vi "Zad2.vi"() -> ()   [LabVIEW 2017]
uses:
  <vilib>/sound2/lvsound2.llb/Sound Data Format.ctl
  Lab 6 - 9.04.2018/mainVIs/States.ctl
  <vilib>/sound2/lvsound2.llb/Sound Input Task ID.ctl
  main VIs/UIData.ctl
  <vilib>/sound2/lvsound2.llb/Sampling Mode.ctl
  <vilib>/measure/maspectr.llb/FFT Power Spectrum and PSD for N Chan.vi
  <vilib>/sound2/lvsound2.llb/Sound Input Read (DBL).vi
  <vilib>/measure/NI_MAPro.lvlib
panel:
  out "Waveform Graph":cluster{"f0":dbl, "df":dbl, "magnitude":dbl[]}[](graph)
  in  "Stop":bool
  in  "Play":bool
  in  "sound format":T1={"sample rate (S/s)"=22050.0, "number of channels"=2, "bits per sample"=16}
  in  "number of samples/ch":i32=100000
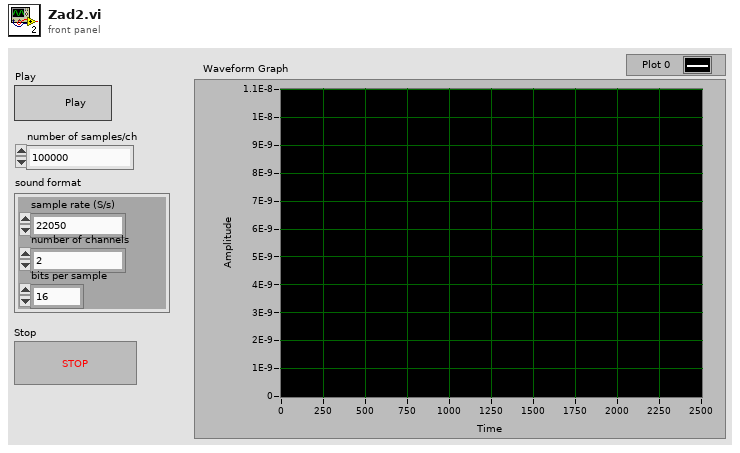
[diagram p1: front panel]
types:
  T1 = typedef "Sound Data Format.ctl" = cluster{"sample rate (S/s)":dbl, "number of channels":i32, "bits per sample":i32}
  T2 = typedef "Sound Input Task ID.ctl" = u32
  T3 = typedef "States.ctl" = enum16{"Idle", "Initialization", "Acquisition", "Finish"}
  T4 = typedef "UIData.ctl" = cluster{"Play":bool, "number of samples/ch":i32, "sound format":T1}
  T5 = typedef "Sampling Mode.ctl" = i32
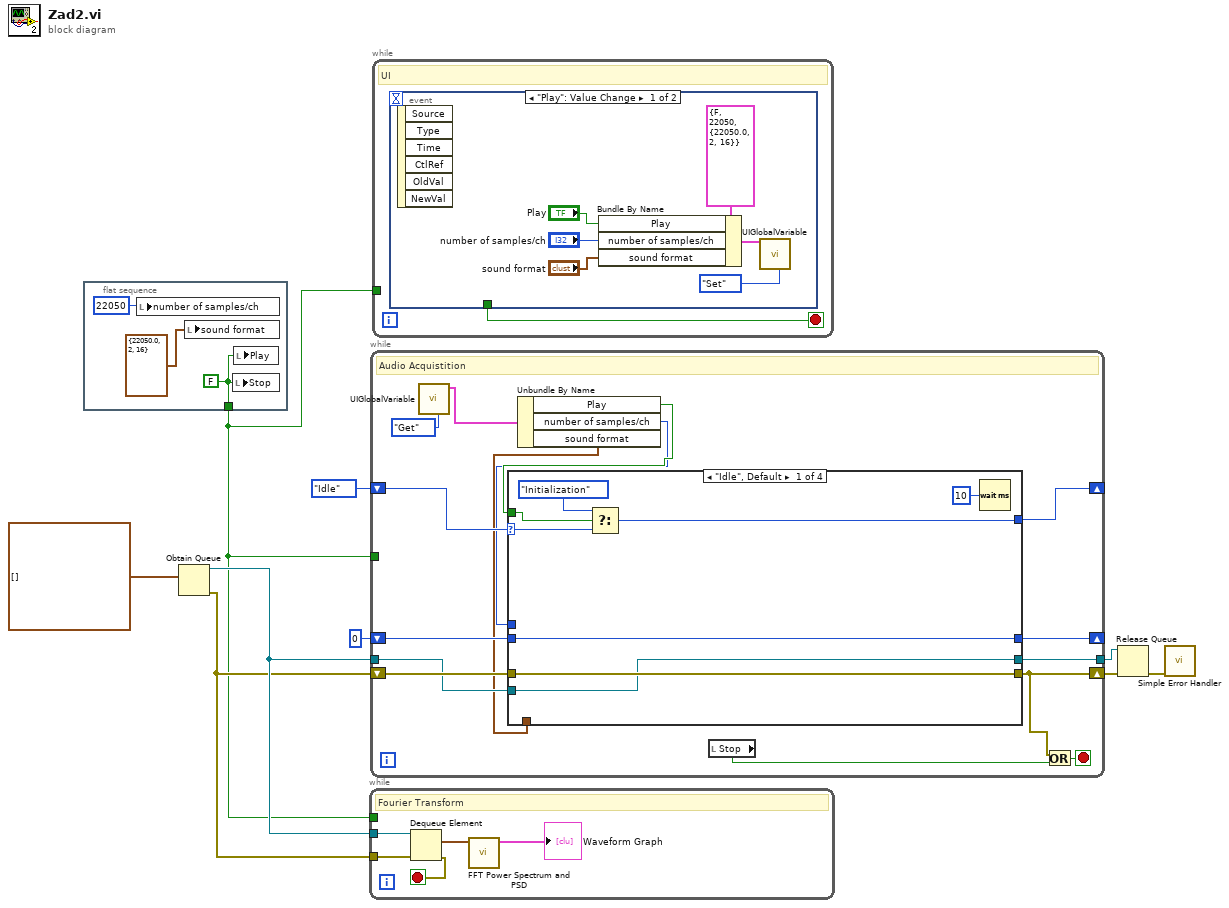
[diagram p0: block diagram]
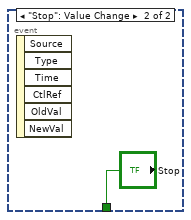
[diagram p2: hidden frame]
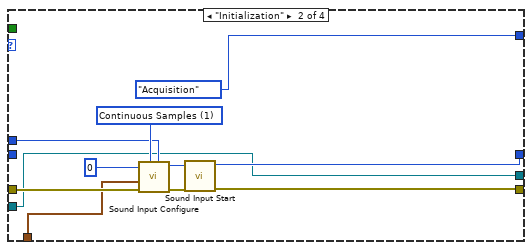
[diagram p3: hidden frame]
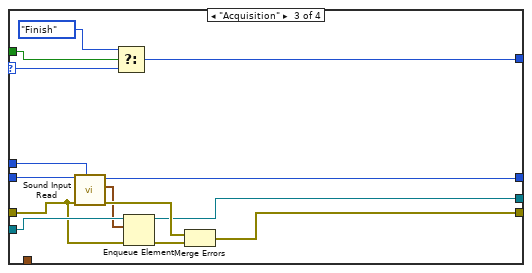
[diagram p4: hidden frame]
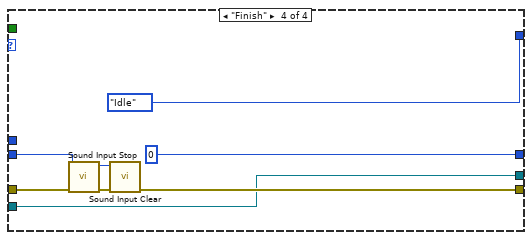
[diagram p5: hidden frame]
diagram:
  n1 = flat-sequence {
    tunnel: [w10] -> w1
    frame #0 {
      w10 = FALSE ("stop")
      n2 = local write "number of samples/ch"(22050 ("number of samples/ch")) -> ()
      n3 = local write "sound format"(T1 {"sample rate (S/s)"=22050.0, "number of channels"=2, "bits per sample"=16} ("sound format")) -> ()
      n4 = local write "Stop"(w10) -> ()
      n5 = local write "Play"(w10) -> ()
    }
  }
  n6 = Obtain Queue(element data type=waveform(dbl)[] [] ("data")) -> (queue out=w4:refnum<queue>, error out=w3:errorcluster)  [unwired: 4 in, 1 out]
  n7 = while {
    tunnel: w4 -> [w17]
    tunnel: w3 -> [w16]
    tunnel: w1 -> [_]
    stop <- w15 stop-if-true
    # "Fourier Transform"
    n8 = Dequeue Element(queue=w17, error in (no error)=w16) -> (element=w14:waveform(dbl)[], error out=w15:errorcluster)  [unwired: 1 in, 2 out]
    n9 = call-poly <vilib>:"FFT Power Spectrum and PSD.vi"("time signals"=w14) -> ("Power Spectrum / PSD"=→"Waveform Graph":cluster{"f0":dbl, "df":dbl, "magnitude":dbl[]}[])  [unwired: 7 in, 3 out]
  }
  n10 = while {
    shift-right: [w31] -> _
    shift-left: States."Idle" ("Enum") -> [w32]
    shift-right: [w26] -> w6
    shift-left: w3 -> [w30]
    shift-right: [w29] -> _
    shift-left: T2 0 ("task ID out") -> [w28]
    tunnel: w1 -> [_]
    tunnel: w4 -> [w25]
    tunnel: [w24] -> w7
    stop <- w27 stop-if-true
    # "Audio Acquistition"
    n11 = call "UIGlobalVariable.vi"("Enum"=enum16{"Get", "Set"}."Get") -> ("Output"=w21:T4)  [unwired: 10 in]
    n12 = Unbundle By Name(w21) -> ("Play"=w20:bool, "number of samples/ch"=w19:i32, "sound format"=w18:T1)
    n13 = case shown="\"Idle\", Default" w32 {
      selector: w32 -> [w37 _ w61 _]
      tunnel: [w40 States."Acquisition" ("Enum") w65 States."Idle" ("Enum")] -> w31
      tunnel: w20 -> [w38 _ w59 _]
      tunnel: [w35 w44 w54 w68] -> w26
      tunnel: w30 -> [w35 w50 w57 w71]
      tunnel: w18 -> [_ w49 _ _]
      tunnel: w19 -> [_ w47 w62 _]
      tunnel: [w36 w43 w63 T2 0 ("task ID out")] -> w29
      tunnel: w28 -> [w36 _ w64 w72]
      tunnel: w25 -> [w34 w41 w58 w66]
      tunnel: [w34 w41 w53 w66] -> w24
      frame "Idle", Default {
        n14 = Select(t=States."Initialization" ("Enum"), s=w38, f=w37) -> (s? t:f=w40:T3)
        n15 = Wait (ms)(milliseconds to wait=u32 10) -> ()  [unwired: 1 out]
      }
      frame "Initialization" {
        w48 = T5 1 items=["Finite Samples", "Continuous Samples"] ("sample mode")
        n16 = call <vilib>:"Sound Input Configure.vi"("number of samples/ch"=w47, "sample mode"=w48, "error in (no error)"=w50, "sound format"=w49, "device ID"=u32 0) -> ("error out"=w45:errorcluster, "task ID"=w46:T2)  [unwired: 5 in]
        n17 = call <vilib>:"Sound Input Start.vi"("error in (no error)"=w45, "task ID"=w46) -> ("error out"=w44:errorcluster, "task ID out"=w43:T2)  [unwired: 8 in]
      }
      frame "Acquisition" {
        n18 = call-poly <vilib>:"Sound Input Read.vi"("number of samples/ch"=w62, "error in (no error)"=w57, "task ID"=w64) -> ("error out"=w55:errorcluster, "data"=w52:waveform(dbl)[], "task ID out"=w63:T2)  [unwired: 6 in]
        n19 = Select(t=States."Finish" ("Enum"), s=w59, f=w61) -> (s? t:f=w65:T3)
        n20 = Enqueue Element(queue=w58, element=w52, error in (no error)=w57) -> (queue out=w53:refnum<queue>, error out=w56:errorcluster)  [unwired: 1 in, 1 out]
        n21 = Merge Errors(w55, w56) -> (w54:errorcluster)
      }
      frame "Finish" {
        n22 = call <vilib>:"Sound Input Stop.vi"("error in (no error)"=w71, "task ID"=w72) -> ("error out"=w69:errorcluster, "task ID out"=w70:T2)  [unwired: 8 in]
        n23 = call <vilib>:"Sound Input Clear.vi"("error in (no error)"=w69, "task ID"=w70) -> ("error out"=w68:errorcluster)  [unwired: 9 in]
      }
    }
    n24 = local read "Stop"() -> (w23:bool)
    n25 = Or(x=w26, y=w23) -> (x .or. y?=w27:bool)
  }
  n26 = while {
    tunnel: w1 -> [_]
    stop <- w74 stop-if-true
    # "UI"
    n27 = event shown="[0] \"Play\": Value Change" {
      selector: _ -> [_ _]
      dyn-events: _ -> [_ _]
      timeout: _ -> [_ _]
      tunnel: [_ "Stop"] -> w74
      event "Play": Value Change {
        n28 = event-data() -> ()  [unwired: 1 in, 6 out]
        n29 = Bundle By Name(cluster=T4 {"Play"=FALSE, "number of samples/ch"=22050, "sound format"={"sample rate (S/s)"=22050.0, "number of channels"=2, "bits per sample"=16}} ("Output"), "Play"="Play", "number of samples/ch"="number of samples/ch", "sound format"="sound format") -> (w80:T4)
        n30 = call "UIGlobalVariable.vi"("Enum"=enum16{"Get", "Set"}."Set", "Input"=w80) -> ()  [unwired: 9 in, 1 out]
      }
      event "Stop": Value Change {
        n31 = event-data() -> ()  [unwired: 1 in, 6 out]
      }
    }
  }
  n32 = Release Queue(queue=w7, error in (no error)=w6) -> (error out=w5:errorcluster)  [unwired: 1 in, 2 out]
  n33 = call <vilib>:"Simple Error Handler.vi"("error in (no error)"=w5) -> ()  [unwired: 4 in, 5 out]
